vi "Execute Update Module Interface.vi"(6 "Mouse Position":T1, 8 "User VI Ref":refnum<vi>, 9 "Menu Item Tag Suffix":string, 10 "Remaining Items":refnum<vi>[](array[refnum]), 11 "Affected Items":T2) -> (0 "Fail transaction?":bool)   [LabVIEW 2025]
doc: "This VI is part of a plug-in for modifying the LabVIEW shortcut menus. This is the execute VI which is called when the shortcut menu is chosen by the user. It performs the action of the selected menu item."
uses:
  Update Module Interface.ctl
  <vilib>/Utility/miscctls.llb/LVPositionTypeDef.ctl
  <vilib>/Utility/traverseref.llb/TRef TravTarget.ctl
  <vilib>/Utility/miscctls.llb/LVPointTypeDef.ctl
  <vilib>/Utility/Data Type/Type Definitions/Data Type.ctl
  <vilib>/Utility/error.llb/Trim Whitespace One-Sided.vi
  <vilib>/Utility/Data Type/NI_Data Type.lvlib
panel:
  # "All controls on this panel except \"Affected Items\" have been locked to prevent accidental edits. Changing the control names or types, other than the elements of the \"Affected Items\" cluster will make the VI unusable as a menu plugin.\n\nSee Context Help for each control for details about its use."
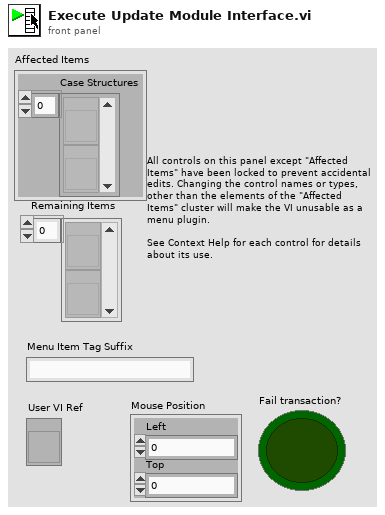
[diagram p1: front panel]
types:
  T1 = typedef "LVPositionTypeDef.ctl" = cluster{"Left":i32, "Top":i32}
  T2 = typedef "Update Module Interface.ctl" = cluster{"Case Structures":refnum<vi>[]}
  T3 = typedef "TRef TravTarget.ctl" = enum16{"FP", "BD", "Other"}
  T4 = typedef "NI_Data Type.lvlib/Data Type.ctl" = enum8{"Invalid Type", "Void", "I8", "I16", "I32", "I64", "U8", "U16", "U32", "U64", "Single Float", "Double Float", "Extended Float", "Single Complex", "Double Complex", "Extended Complex", "Enum U8", "Enum U16", "Enum U32", "Enum U64", "Single Float With Unit", "Double Float With Unit", "Extended Float With Unit", "Single Complex with Unit", "Double Complex with Unit", "Extended Complex with Unit", "Boolean", "String", "Path", "Picture", "Tag", "Array", "Cluster", "Variant", "LV Variant", "Waveform", "Timestamp", "Digital Waveform", "Digital Data", "ExpressData", "Refnum", "External Data", "VI", "Poly VI", "LabVIEW Class Instance", "Fixed Point", "Set Collection", "Map Collection"}
  T5 = typedef "LVPointTypeDef.ctl" = cluster{"Horizontal":i16, "Vertical":i16}
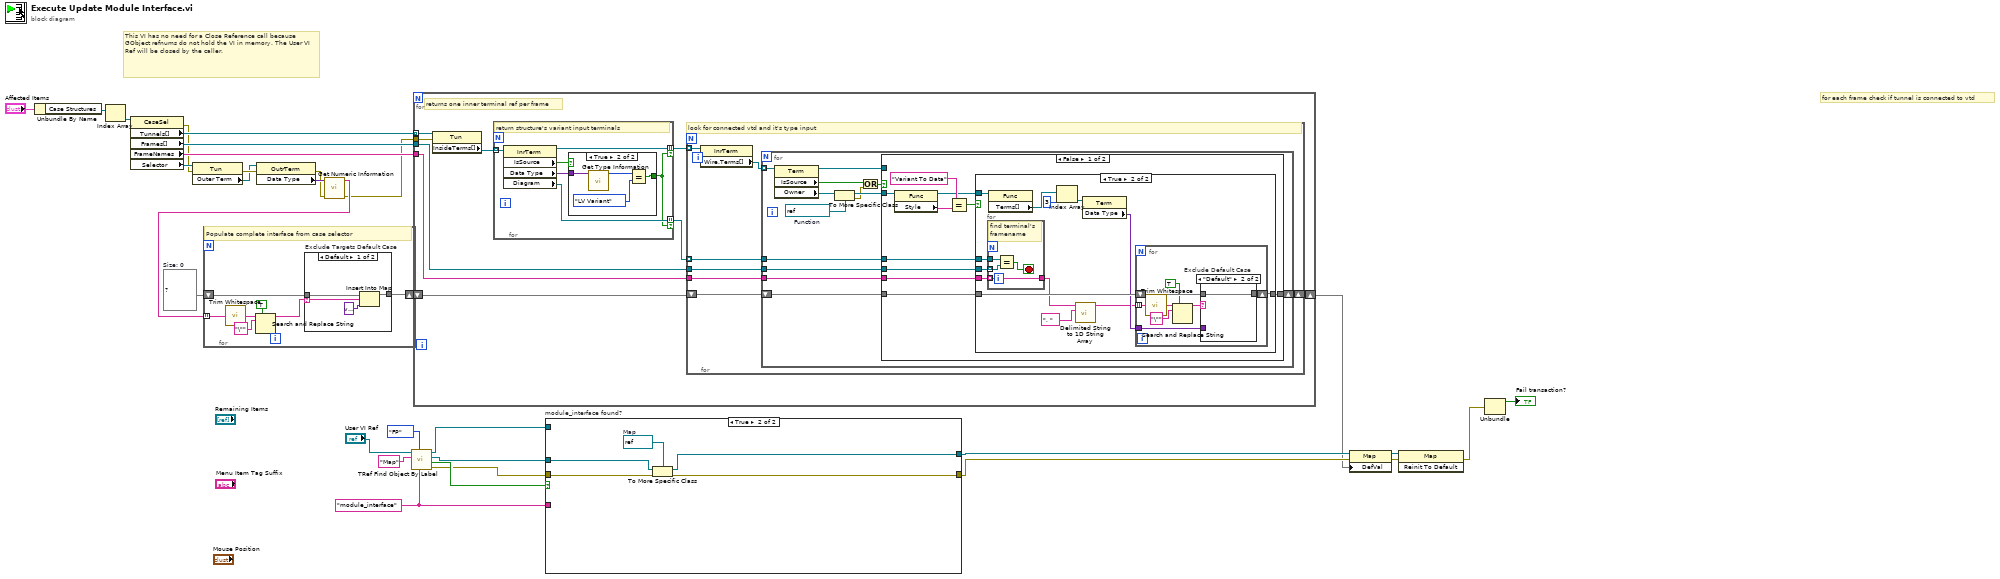
[diagram p0: block diagram]
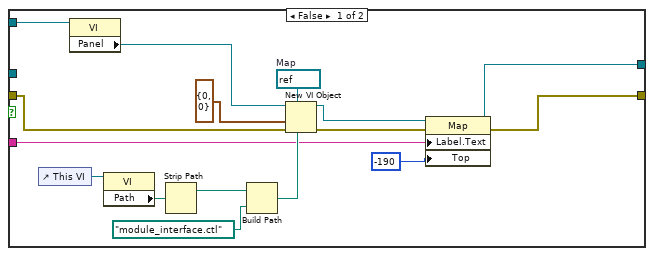
[diagram p3: hidden frame]
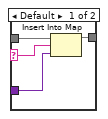
[diagram p6: hidden frame]
diagram:
  w15 = "module_interface" ("y")
  w11 = map{string, variant} {}  # Size: 0
  # "for each frame check if tunnel is connected to vtd"
  # "This VI has no need for a Close Reference call because GObject refnums do not hold the VI in memory. The User VI Ref will be closed by the caller."
  n1 = Unbundle By Name("Affected Items") -> ("Case Structures"=w30:refnum<vi>[])
  n2 = Index Array(array=w30) -> (element=w29:refnum<vi>)  [unwired: 1 in]
  n3 = property class="CaseSel"(reference=w29) -> (error out=w6:errorcluster, "Tunnels[]"=w28:refnum<vi>[], "Frames[]"=w27:refnum<vi>[], "FrameNames"=w10:string[], "Selector"=w8:refnum<vi>)  [unwired: 1 in, 1 out]
  n4 = property class="Tun"(reference=w8, error in=w6) -> (error out=w7:errorcluster, "Outer Term"=w5:refnum<vi>)  [unwired: 1 out]
  n5 = property class="OutrTerm"(reference=w5, error in=w7) -> (error out=w3:errorcluster, "Data Type"=w4:variant)  [unwired: 1 out]
  n6 = call <vilib>:"Get Numeric Information.vi"("error in (no error)"=w3, "variant"=w4) -> ("error out"=w1:errorcluster, "enum names"=w2:string[])  [unwired: 6 in, 2 out]
  n7 = for {
    shift-right: [w37] -> w9
    shift-left: w11 -> [w38]
    tunnel: w2 -> [w33] mode=indexing
    # "Populate complete interface from case selector"
    n8 = call <vilib>:"Trim Whitespace.vi"("string"=w33) -> ("trimmed string"=w34:string)  [unwired: 1 in]
    n9 = Search and Replace String(replace all?=TRUE ("replace all? (F)"), input string=w34, search string="\"") -> (result string=w32:string)  [unwired: 5 in, 3 out]
    n10 = case "Exclude Targets Default Case" shown="Default" w32 {
      selector: w32 -> [w40 _]
      tunnel: w38 -> [w42 w43]
      tunnel: [w41 w43] -> w37
      frame Default {
        n11 = Insert Into Map(map in=w42, key=w40, value=variant) -> (map out=w41:map{string, variant})  [unwired: 2 out]
      }
      frame "Default" {
      }
    }
  }
  n12 = call <vilib>:"TRef Find Object By Label.vi"("Label"=w15, "Traverse Target"=TRef_TravTarget."FP", "Class Name"="Map", "VI Ref"="User VI Ref") -> ("error out"=w18:errorcluster, "Found?"=w19:bool, "Found Obj Ref"=w17:refnum<vi>, "dup VI Ref"=w16:refnum<vi>)  [unwired: 4 in]
  n13 = for {
    tunnel: w28 -> [w52] mode=indexing
    tunnel: w27 -> [w49]
    tunnel: w10 -> [w48]
    shift-right: [w46] -> w14
    shift-left: w9 -> [w45]
    tunnel: w1 -> [w44]
    # "returns one inner terminal ref per frame"
    n14 = property class="Tun"(reference=w52, error in=w44) -> ("InsideTerms[]"=w51:refnum<vi>[])  [unwired: 2 out]
    n15 = for {
      tunnel: w51 -> [w58] mode=indexing
      tunnel: [w57] -> w50 mode=indexing if=w53
      tunnel: [w54] -> w47 mode=indexing if=w53
      # "return structure's variant input terminals"
      n16 = property class="InrTerm"(reference=w58) -> (reference out=w57:refnum<vi>, "IsSource"=w55:bool, "Data Type"=w56:variant, "Diagram"=w54:refnum<vi>)  [unwired: 1 in, 1 out]
      n17 = case shown="True" w55 {
        selector: w55 -> [w59 _]
        tunnel: w56 -> [_ w63]
        tunnel: [w59 w60] -> w53
        frame False {
        }
        frame True {
          n18 = call <vilib>:"Get Type Information.vi"("variant"=w63) -> ("type"=w61:T4)  [unwired: 6 in, 4 out]
          n19 = Equal?(x=w61, y=Data_Type."LV Variant" ("type")) -> (x = y?=w60:bool)
        }
      }
    }
    n20 = for {
      tunnel: w50 -> [w69] mode=indexing
      tunnel: w49 -> [w68]
      tunnel: w48 -> [w67]
      tunnel: w47 -> [w66] mode=indexing
      shift-right: [w64] -> w46
      shift-left: w45 -> [w65]
      # "look for connected vtd and it's type input"
      n21 = property class="InrTerm"(reference=w69) -> ("Wire.Terms[]"=w70:refnum<vi>[])  [unwired: 1 in, 2 out]
      n22 = for {
        tunnel: w70 -> [w83] mode=indexing
        tunnel: w68 -> [w75]
        tunnel: w67 -> [w74]
        tunnel: w66 -> [w73]
        shift-right: [w71] -> w64
        shift-left: w65 -> [w72]
        w78 = refnum<vi> refnum  # Function
        n23 = property class="Term"(reference=w83) -> (reference out=w81:refnum<vi>, "IsSource"=w82:bool, "Owner"=w80:refnum<vi>)  [unwired: 1 in, 1 out]
        n24 = To More Specific Class(target class=w78, reference=w80) -> (specific class reference=w79:refnum<vi>, error out=w76:errorcluster)  [unwired: 1 in]
        n25 = Or(x=w82, y=w76) -> (x .or. y?=w77:bool)
        n26 = case shown="False" w77 {
          tunnel: w81 -> [_ _]
          tunnel: w79 -> [w93 _]
          tunnel: w75 -> [w88 _]
          tunnel: w74 -> [w87 _]
          tunnel: w73 -> [w86 _]
          tunnel: w72 -> [w85 w125]
          tunnel: [w84 w125] -> w71
          frame False {
            n27 = property class="Func"(reference=w93) -> (reference out=w89:refnum<vi>, "Style"=w92:string)  [unwired: 1 in, 1 out]
            n28 = Equal?(x="Variant To Data", y=w92) -> (x = y?=w90:bool)
            n29 = case shown="True" w90 {
              tunnel: w89 -> [_ w104]
              tunnel: w88 -> [_ w103]
              tunnel: w87 -> [_ w102]
              tunnel: w86 -> [_ w101]
              tunnel: w85 -> [w94 w100]
              tunnel: [w94 w98] -> w84
              frame False {
              }
              frame True {
                n30 = for {
                  tunnel: w103 -> [w124] mode=indexing
                  tunnel: w102 -> [w123] mode=indexing
                  tunnel: [w123] -> w97
                  tunnel: w101 -> [w121]
                  stop <- w122 stop-if-true
                  # "find terminal's\nframename"
                  n31 = Equal?(x=w121, y=w124) -> (x = y?=w122:bool)
                }
                n32 = property class="Func"(reference=w104) -> ("Terms[]"=w107:refnum<vi>[])  [unwired: 1 in, 2 out]
                n33 = Index Array(array=w107, index=3) -> (element=w105:refnum<vi>)
                n34 = call <vilib>:"Delimited String to 1D String Array.vi"("delimiter"=", ", "delimited string"=w97) -> ("string array"=w95:string[])  [unwired: 9 in]
                n35 = property class="Term"(reference=w105) -> ("Data Type"=w99:variant)  [unwired: 1 in, 2 out]
                n36 = for {
                  tunnel: w99 -> [w114]
                  tunnel: w95 -> [w109] mode=indexing
                  shift-right: [w113] -> w98
                  shift-left: w100 -> [w115]
                  n37 = call <vilib>:"Trim Whitespace.vi"("string"=w109) -> ("trimmed string"=w108:string)  [unwired: 1 in]
                  n38 = Search and Replace String(replace all?=TRUE ("replace all? (F)"), input string=w108, search string="\"") -> (result string=w110:string)  [unwired: 5 in, 3 out]
                  n39 = case "Exclude Default Case" shown="\"Default\"" w110 {
                    selector: w110 -> [w116 _]
                    tunnel: w115 -> [w119 w120]
                    tunnel: [w118 w120] -> w113
                    tunnel: w114 -> [w117 _]
                    frame Default {
                      n40 = Insert Into Map(map in=w119, key=w116, value=w117) -> (map out=w118:map{string, variant})  [unwired: 2 out]
                    }
                    frame "Default" {
                    }
                  }
                }
              }
            }
          }
          frame True {
          }
        }
      }
    }
  }
  n41 = case "module_interface found?" shown="True" w19 {
    tunnel: [w128 w143] -> w24
    tunnel: w17 -> [_ w144]
    tunnel: [w130 w146] -> w23
    tunnel: w15 -> [w127 _]
    tunnel: w16 -> [w139 _]
    tunnel: w18 -> [w138 w145]
    frame False {
      w136 = refnum<vi> refnum  # Map
      n42 = control-ref of="This VI"() -> (w135:refnum<vi>)
      n43 = property class="VI"(reference=w139) -> ("Panel"=w137:refnum<vi>)  [unwired: 1 in, 2 out]
      n44 = property class="VI"(reference=w135) -> ("Path"=w134:path)  [unwired: 1 in, 2 out]
      n45 = Strip Path(path=w134) -> (stripped path=w132:path)  [unwired: 1 out]
      n46 = Build Path(base path=w132, name or relative path=path "module_interface.ctl") -> (appended path=w133:path)
      n47 = New VI Object(vi object class=w136, owner refnum=w137, position/next to=T5 {"Horizontal"=0, "Vertical"=0} ("location"), 6:w133, 8:w138) -> (object refnum=w129:refnum<vi>, 0:w140:errorcluster)  [unwired: 3 in]
      n48 = property class="Map"(reference=w129, error in=w140, "Label.Text"=w127, "Top"=-190 ("Position:Top")) -> (reference out=w128:refnum<vi>, error out=w130:errorcluster)
    }
    frame True {
      w142 = refnum<vi> refnum  # Map
      n49 = To More Specific Class(target class=w142, reference=w144, error in=w145) -> (specific class reference=w143:refnum<vi>, error out=w146:errorcluster)
    }
  }
  n50 = property class="Map"(reference=w24, error in=w23, "DefVal"=w14) -> (reference out=w12:refnum<vi>, error out=w25:errorcluster)
  n51 = invoke class="Map" method="Reinit To Default"(reference=w12, error in=w25) -> (error out=w13:errorcluster)  [unwired: 1 in, 2 out]
  n52 = Unbundle(w13) -> ("status"=→"Fail transaction?":bool)  [unwired: 2 out]
